vi "EnableDisableButtons.vi"(7 "Action":T1(ring), 8 "ErrorArray In":errorcluster[](array[cluster])) -> (0 "ErrorArray Out":errorcluster[](array[cluster]))   [LabVIEW 2017, in "Framework.lvlib"]
uses:
  Framework.lvlib
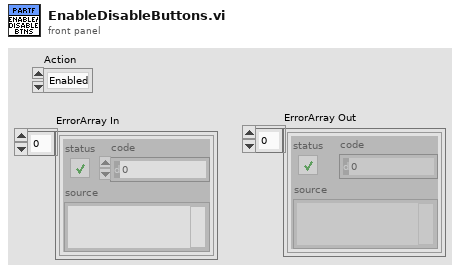
[diagram p1: front panel]
types:
  T1 = enum8{"Enabled", "Disabled", "Disabled and Grayed Out"}
  T2 = typedef "Framework.lvlib/clFrontPanelButtonRefs.ctl" = cluster{"SaveRef":refnum<vi>, "SingleRunRef":refnum<vi>, "MonteCarloRef":refnum<vi>, "AppConfigRef":refnum<vi>, "chkScriptWindowRef":refnum<vi>, "btnOutToFileConfig":refnum<vi>, "AppTypeRef":refnum<vi>, "chkShowPanel":refnum<vi>}
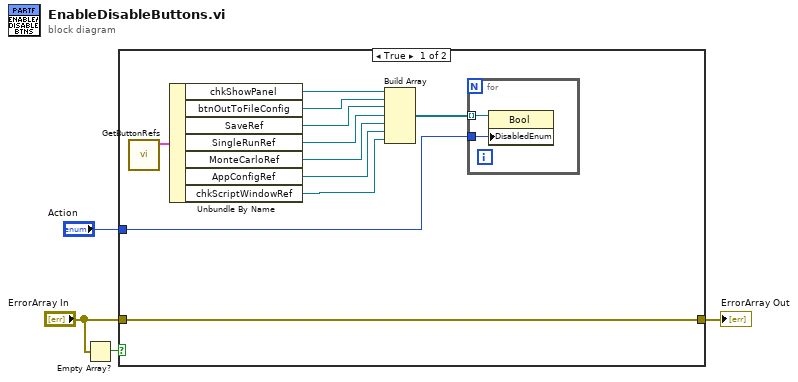
[diagram p0: block diagram]
diagram:
  n1 = Empty Array?(array="ErrorArray In") -> (empty?=w2:bool)
  n2 = case shown="True" w2 {
    tunnel: [w5 w18] -> w4
    tunnel: "ErrorArray In" -> [w5 w18]
    tunnel: "Action" -> [w7 _]
    frame True {
      n3 = call "GetButtonRefs.vi"() -> ("BtnRefs"=w8:T2)  [unwired: 11 in]
      n4 = Unbundle By Name(w8) -> ("chkShowPanel"=w9:refnum<vi>, "btnOutToFileConfig"=w10:refnum<vi>, "SaveRef"=w15:refnum<vi>, "SingleRunRef"=w14:refnum<vi>, "MonteCarloRef"=w13:refnum<vi>, "AppConfigRef"=w12:refnum<vi>, "chkScriptWindowRef"=w11:refnum<vi>)
      n5 = Build Array(w9, w10, w15, w14, w13, w12, w11) -> (w6:refnum<vi>[])
      n6 = for {
        tunnel: w6 -> [w17] mode=indexing
        tunnel: w7 -> [w16]
        n7 = property class="Bool"(reference=w17, "DisabledEnum"=w16) -> ()  [unwired: 1 in, 2 out]
      }
    }
    frame False {
    }
  }
  "ErrorArray Out" <- w4
